vi "Voltage measurment on multimeter.vi"(8 "error in (no error)":errorcluster, 10 "Function (0: DC Volts) 2":u16(ring)=1 items=["DC Volts", "AC Volts", "DC Current", "AC Current", "2-Wire Resistance", "4-Wire Resistance"], 11 "VISA resource name 3":refnum<visa-resource-name>="USB0::0x1AB1::0x0C94::DM3O194400985::INSTR") -> (0 "error out":errorcluster, 1 "Minimum":dbl, 2 "Average":dbl, 3 "Maximum":dbl, 5 "Instantaneous":dbl)   [LabVIEW 2018]
uses:
  <instrlib>/RIGOL DM3058/RIGOL DM3058.lvlib
panel:
  in  "Absolute Resolution (0: 5.5 Rate:Slow)":u16(ring)=2 items=["5.5 Rate:Slow", "4.5 Rate:Middle", "4.5 Rate:Fast", "3.5 Rate", "6.5 Rate"]
  in  "Manual Range (1.0) 2":dbl=1.0
  in  "Auto Range (T: Enable) 2":bool=TRUE
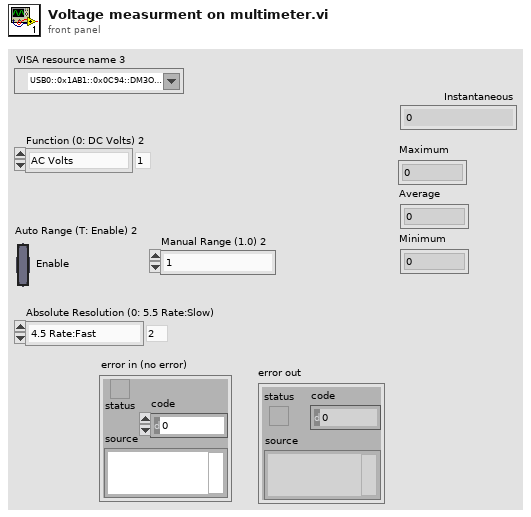
[diagram p1: front panel]
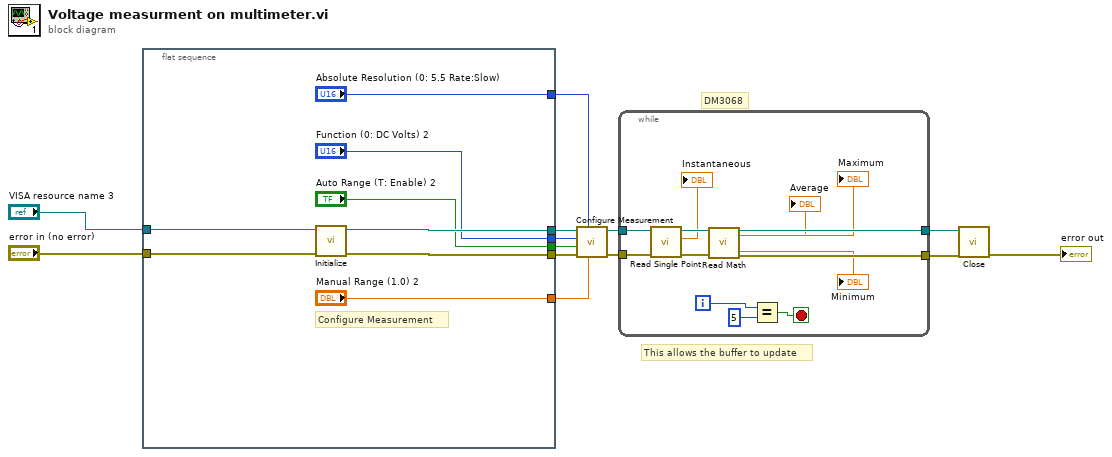
[diagram p0: block diagram]
diagram:
  # "This allows the buffer to update"
  # "DM3068"
  n1 = flat-sequence {
    tunnel: [w21] -> w7
    tunnel: [w20] -> w8
    tunnel: ["Function (0: DC Volts) 2"] -> w9
    tunnel: ["Manual Range (1.0) 2"] -> w10
    tunnel: ["Auto Range (T: Enable) 2"] -> w11
    tunnel: "VISA resource name 3" -> [w16]
    tunnel: "error in (no error)" -> [w15]
    tunnel: ["Absolute Resolution (0: 5.5 Rate:Slow)"] -> w3
    frame #0 {
      # "Configure Measurement"
      n2 = call <instrlib>:"Initialize.vi"("error in (no error)"=w15, "VISA resource name"=w16) -> ("error out"=w20:errorcluster, "VISA resource name out"=w21:refnum<visa-resource-name>)  [unwired: 3 in, 5 out]
    }
  }
  n3 = call <instrlib>:"Configure Measurement.vi"("Manual Range (1.00)"=w10, "Absolute Resolution (0: 5.5 Rate:Slow)"=w3, "error in (no error)"=w8, "Auto Range (T:Enable)"=w11, "Function (0: DC Volts)"=w9, "VISA resource name"=w7) -> ("error out"=w12:errorcluster, "VISA resource name out"=w13:refnum<visa-resource-name>)  [unwired: 4 out]
  n4 = while {
    tunnel: w13 -> [w34]
    tunnel: w12 -> [w33]
    tunnel: [w27] -> w2
    tunnel: [w26] -> w1
    i -> [w30]
    stop <- w32 stop-if-true
    n5 = call <instrlib>:"Read Single Point.vi"("error in (no error)"=w33, "VISA resource name"=w34) -> ("error out"=w28:errorcluster, "Measurement"=→"Instantaneous":dbl, "VISA resource name out"=w29:refnum<visa-resource-name>)  [unwired: 7 out]
    n6 = call <instrlib>:"Read Math.vi"("VISA resource name"=w29, "error in (no error)"=w28) -> ("Maximum"=→"Maximum":dbl, "Average"=→"Average":dbl, "VISA resource name out"=w27:refnum<visa-resource-name>, "Minimum"=→"Minimum":dbl, "error out"=w26:errorcluster)  [unwired: 5 in, 4 out]
    n7 = Equal?(x=w30, y=u32 5) -> (x = y?=w32:bool)
  }
  n8 = call <instrlib>:"Close.vi"("error in (no error)"=w1, "VISA resource name"=w2) -> ("error out"=→"error out":errorcluster)  [unwired: 9 out]
